vi "XML To Experiment Data.vi"(1 "XML Data":string) -> (0 "Experiment Data":T1)   [LabVIEW 2013]
uses:
  Types/Experiment Data.ctl
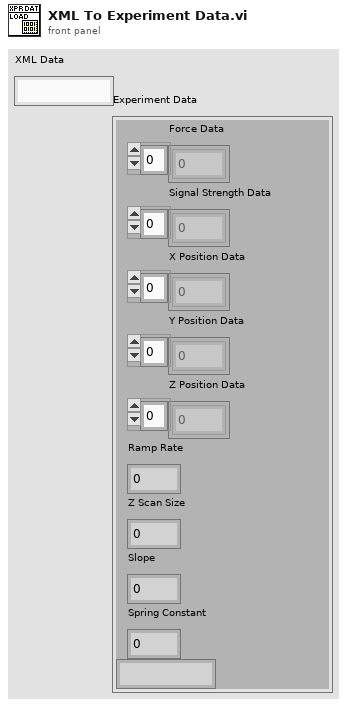
[diagram p1: front panel]
types:
  T1 = typedef "Experiment Data.ctl" = cluster{"Force Data":dbl[], "Signal Strength Data":dbl[], "X Position Data":dbl[], "Y Position Data":dbl[], "Z Position Data":dbl[], "Ramp Rate":dbl, "Z Scan Size":dbl, "Slope":dbl, "Spring Constant":dbl, "Version":string}
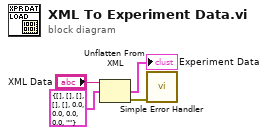
[diagram p0: block diagram]
diagram:
  n1 = Unflatten From XML(xml string="XML Data", type=T1 {"Force Data"=[], "Signal Strength Data"=[], "X Position Data"=[], "Y Position Data"=[], "Z Position Data"=[], "Ramp Rate"=0.0, "Z Scan Size"=0.0, "Slope"=0.0, "Spring Constant"=0.0, "Version"=""} ("Default Experiment Serialized Data")) -> (value=→"Experiment Data":T1, error out=w3:errorcluster)  [unwired: 1 in]
  n2 = call <vilib>:"Simple Error Handler.vi"("error in (no error)"=w3) -> ()  [unwired: 4 in, 5 out]
